vi "Move Home Impl.vi"(8 "error in (no error)":errorcluster, 11 "Ludl Stage in":refnum<class "Ludl Stage.lvclass">) -> (0 "error out":errorcluster, 3 "Ludl Stage out":refnum<class "Ludl Stage.lvclass">)   [LabVIEW 2023, in "Ludl Stage.lvlib" / "Ludl Stage.lvclass"]
uses:
  Ludl Stage.lvclass
  Ludl Stage.lvclass/Ludl Stage.ctl
  Stage Controller/Stage Controller.lvclass
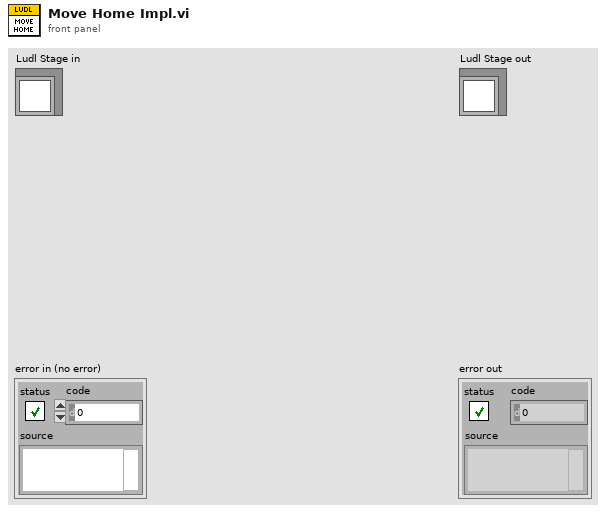
[diagram p1: front panel]
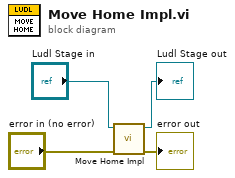
[diagram p0: block diagram]
diagram:
  n1 = call-parent "Move Home Impl.vi"("error in (no error)"="error in (no error)", "Stage Controller in"="Ludl Stage in") -> ("error out"=→"error out":errorcluster, "Stage Controller out"=→"Ludl Stage out":refnum<class "Ludl Stage.lvclass">)  [unwired: 8 in]
